vi "输入数据解析.vi"(0 "单个参数补充":dbl, 1 "从板号":dbl=1.0, 2 "主板二维码":string="BNET01", 3 "从板二维码":string="BNET01", 5 "主板引用":refnum<vi>, 7 "从板引用":refnum<vi>, 9 "主板选项":string="三级故障阀值", 11 "枚举":enum16{"主板", "从板"}(ring), 12 "快换":bool caption="快换写入") -> (4 "输出数组":dbl[][](array[numeric]), 6 "数组长度":dbl[](array[numeric]), 8 "循环次数":i32, 10 "命令":u32, 14 "名称":string[](array[string]), 15 "命令序号":u32[](array[numeric]))   [LabVIEW 2013] (continued)
                    n6602 = call "输入分辨率计算-EV05.vi"("1字节?"=FALSE, "数值"=w16869, "分辨率"=0.001) -> ("低字节"=w16871:dbl, "高字节1"=w16872:dbl)  [unwired: 2 in, 5 out]
                  }
                  frame Disabled {
                    w16875 = 255 ("高字节1")
                  }
                }
                n6603 = Build Array(w16868, w16867) -> (w16866:dbl[])
              }
              frame 1 {
                # "电压过低"
                n6604 = disable-structure shown="启用" {
                  disable-tunnel: [w16883 w16886] -> w16879
                  disable-tunnel: [w16882 w16886] -> w16878
                  disable-tunnel: w16876 -> [w16881 _]
                  frame Disabled {
                    n6605 = Unbundle By Name(w16881) -> ("电压过低"=w16880:dbl)
                    n6606 = call "输入分辨率计算-EV05.vi"("1字节?"=FALSE, "数值"=w16880, "分辨率"=0.1) -> ("低字节"=w16882:dbl, "高字节1"=w16883:dbl)  [unwired: 2 in, 5 out]
                  }
                  frame Enabled {
                    w16886 = 255 ("高字节1")
                  }
                }
                n6607 = Build Array(w16879, w16878) -> (w16877:i32[])
              }
              frame 2 {
                # "电压不均衡"
                n6608 = disable-structure shown="启用" {
                  disable-tunnel: [w16894 w16897] -> w16890
                  disable-tunnel: [w16893 w16897] -> w16889
                  disable-tunnel: w16887 -> [w16892 _]
                  frame Disabled {
                    n6609 = Unbundle By Name(w16892) -> ("电压不均衡(V)"=w16891:dbl)
                    n6610 = call "输入分辨率计算-EV05.vi"("1字节?"=FALSE, "数值"=w16891, "分辨率"=0.1) -> ("低字节"=w16893:dbl, "高字节1"=w16894:dbl)  [unwired: 2 in, 5 out]
                  }
                  frame Enabled {
                    w16897 = 255 ("高字节1")
                  }
                }
                n6611 = Build Array(w16890, w16889) -> (w16888:i32[])
              }
              frame 3 {
                # "温度过高"
                n6612 = disable-structure shown="启用" {
                  disable-tunnel: [w16904 255 ("高字节1")] -> w16900
                  disable-tunnel: w16898 -> [w16902 _]
                  frame Disabled {
                    n6613 = Unbundle By Name(w16902) -> ("温度过高"=w16901:dbl)
                    n6614 = call "输入分辨率计算-EV05.vi"("1字节?"=TRUE, "数值"=w16901, "偏移量"=-40.0, "分辨率"=1.0) -> ("高字节1"=w16904:dbl)  [unwired: 1 in, 6 out]
                  }
                  frame Enabled {
                  }
                }
                n6615 = Build Array(w16900) -> (w16899:i32[])
              }
              frame 4 {
                # "温度过低"
                n6616 = disable-structure shown="启用" {
                  disable-tunnel: [w16914 255 ("高字节1")] -> w16910
                  disable-tunnel: w16908 -> [w16912 _]
                  frame Disabled {
                    n6617 = Unbundle By Name(w16912) -> ("温度过低"=w16911:dbl)
                    n6618 = call "输入分辨率计算-EV05.vi"("1字节?"=TRUE, "数值"=w16911, "偏移量"=-40.0, "分辨率"=1.0) -> ("高字节1"=w16914:dbl)  [unwired: 1 in, 6 out]
                  }
                  frame Enabled {
                  }
                }
                n6619 = Build Array(w16910) -> (w16909:i32[])
              }
              frame 5 {
                # "温度不均衡"
                n6620 = disable-structure shown="启用" {
                  disable-tunnel: [w16923 255 ("高字节1")] -> w16920
                  disable-tunnel: w16918 -> [w16922 _]
                  frame Disabled {
                    n6621 = Unbundle By Name(w16922) -> ("温度不均衡"=w16921:dbl)
                    n6622 = call "输入分辨率计算-EV05.vi"("1字节?"=TRUE, "数值"=w16921, "分辨率"=1.0) -> ("高字节1"=w16923:dbl)  [unwired: 2 in, 6 out]
                  }
                  frame Enabled {
                  }
                }
                n6623 = Build Array(w16920) -> (w16919:i32[])
              }
              frame 6 {
                # "SOC过低"
                n6624 = disable-structure shown="启用" {
                  disable-tunnel: w16929 -> [w16946 _]
                  disable-tunnel: [w16932 w16949] -> w16928
                  disable-tunnel: [w16931 w16949] -> w16927
                  frame Disabled {
                    n6625 = Unbundle By Name(w16946) -> ("SOC过低"=w16945:dbl)
                    n6626 = call "输入分辨率计算-EV05.vi"("1字节?"=FALSE, "数值"=w16945, "分辨率"=0.1) -> ("低字节"=w16934:dbl, "高字节1"=w16935:dbl)  [unwired: 2 in, 5 out]
                    n6627 = call "二进制解析-8.6.vi"("索引"=4, "数值"=0) -> ("低位子数组"=w16938:i32[])  [unwired: 3 out]
                    n6628 = call "二进制解析-8.6.vi"("索引"=4, "数值"=w16935) -> ("低位子数组"=w16941:i32[])  [unwired: 3 out]
                    n6629 = call "二进制解析-8.6.vi"("索引"=4, "数值"=w16934) -> ("低位子数组"=w16939:i32[], "高位子数组"=w16940:i32[])  [unwired: 2 out]
                    n6630 = Insert Into Array(array=w16941, new element=w16940) -> (w16943:i32[])  [unwired: 1 in]
                    n6631 = Insert Into Array(array=w16939, new element=w16938) -> (w16937:i32[])  [unwired: 1 in]
                    n6632 = call "数值二进制转十进制-8.6.vi"("子数组"=w16937) -> ("十进制数值"=w16932:i32)  [unwired: 4 out]
                    n6633 = call "数值二进制转十进制-8.6.vi"("子数组"=w16943) -> ("十进制数值"=w16931:i32)  [unwired: 4 out]
                  }
                  frame Enabled {
                    w16949 = 255 ("高字节1")
                  }
                }
                n6634 = Build Array(w16927, w16928) -> (w16930:i32[])
              }
            }
            n6635 = Insert Into Array(array=w16861, new element=w16860) -> (w16862:dbl[])  [unwired: 1 in]
          }
          n6636 = Build Array(w16855) -> (w16854:dbl[][])
        }
        frame "电压过低" {
          n6637 = Unbundle By Name(w16954) -> ("一级故障(从板)"=w16955:refnum<vi>)
          n6638 = property class="Clust (严格)"(reference=w16955) -> ("Value"=w16953:T8)  [unwired: 1 in, 2 out]
          n6639 = for {
            N: 7 -> [_]
            tunnel: w16953 -> [w16965]
            shift-right: [w16964] -> w16957
            shift-left: dbl[] [] -> [w16963]
            i -> [w16966]
            n6640 = case shown="1" w16966 {
              tunnel: w16965 -> [w16967 w16978 w16989 w17000 w17010 w17020 w17031]
              tunnel: [w16968 w16979 w16990 w17001 w17011 w17021 w17032] -> w16962
              frame 0, Default {
                # "电压过高"
                n6641 = disable-structure shown="启用" {
                  disable-tunnel: [w16974 w16977] -> w16970
                  disable-tunnel: [w16973 w16977] -> w16969
                  disable-tunnel: w16967 -> [w16972 _]
                  frame Disabled {
                    n6642 = Unbundle By Name(w16972) -> ("电压过高"=w16971:dbl)
                    n6643 = call "输入分辨率计算-EV05.vi"("1字节?"=FALSE, "数值"=w16971, "分辨率"=0.1) -> ("低字节"=w16973:dbl, "高字节1"=w16974:dbl)  [unwired: 2 in, 5 out]
                  }
                  frame Enabled {
                    w16977 = 255 ("高字节1")
                  }
                }
                n6644 = Build Array(w16970, w16969) -> (w16968:i32[])
              }
              frame 1 {
                # "电压过低"
                n6645 = disable-structure shown="启用" {
                  disable-tunnel: [w16985 w16988] -> w16981
                  disable-tunnel: [w16984 w16988] -> w16980
                  disable-tunnel: w16978 -> [w16983 _]
                  frame Enabled {
                    n6646 = Unbundle By Name(w16983) -> ("电压过低"=w16982:dbl)
                    n6647 = call "输入分辨率计算-EV05.vi"("1字节?"=FALSE, "数值"=w16982, "分辨率"=0.001) -> ("低字节"=w16984:dbl, "高字节1"=w16985:dbl)  [unwired: 2 in, 5 out]
                  }
                  frame Disabled {
                    w16988 = 255 ("高字节1")
                  }
                }
                n6648 = Build Array(w16981, w16980) -> (w16979:dbl[])
              }
              frame 2 {
                # "电压不均衡"
                n6649 = disable-structure shown="启用" {
                  disable-tunnel: [w16996 w16999] -> w16992
                  disable-tunnel: [w16995 w16999] -> w16991
                  disable-tunnel: w16989 -> [w16994 _]
                  frame Disabled {
                    n6650 = Unbundle By Name(w16994) -> ("电压不均衡(V)"=w16993:dbl)
                    n6651 = call "输入分辨率计算-EV05.vi"("1字节?"=FALSE, "数值"=w16993, "分辨率"=0.1) -> ("低字节"=w16995:dbl, "高字节1"=w16996:dbl)  [unwired: 2 in, 5 out]
                  }
                  frame Enabled {
                    w16999 = 255 ("高字节1")
                  }
                }
                n6652 = Build Array(w16992, w16991) -> (w16990:i32[])
              }
              frame 3 {
                # "温度过高"
                n6653 = disable-structure shown="启用" {
                  disable-tunnel: [w17006 255 ("高字节1")] -> w17002
                  disable-tunnel: w17000 -> [w17004 _]
                  frame Disabled {
                    n6654 = Unbundle By Name(w17004) -> ("温度过高"=w17003:dbl)
                    n6655 = call "输入分辨率计算-EV05.vi"("1字节?"=TRUE, "数值"=w17003, "偏移量"=-40.0, "分辨率"=1.0) -> ("高字节1"=w17006:dbl)  [unwired: 1 in, 6 out]
                  }
                  frame Enabled {
                  }
                }
                n6656 = Build Array(w17002) -> (w17001:i32[])
              }
              frame 4 {
                # "温度过低"
                n6657 = disable-structure shown="启用" {
                  disable-tunnel: [w17016 255 ("高字节1")] -> w17012
                  disable-tunnel: w17010 -> [w17014 _]
                  frame Disabled {
                    n6658 = Unbundle By Name(w17014) -> ("温度过低"=w17013:dbl)
                    n6659 = call "输入分辨率计算-EV05.vi"("1字节?"=TRUE, "数值"=w17013, "偏移量"=-40.0, "分辨率"=1.0) -> ("高字节1"=w17016:dbl)  [unwired: 1 in, 6 out]
                  }
                  frame Enabled {
                  }
                }
                n6660 = Build Array(w17012) -> (w17011:i32[])
              }
              frame 5 {
                # "温度不均衡"
                n6661 = disable-structure shown="启用" {
                  disable-tunnel: [w17025 255 ("高字节1")] -> w17022
                  disable-tunnel: w17020 -> [w17024 _]
                  frame Disabled {
                    n6662 = Unbundle By Name(w17024) -> ("温度不均衡"=w17023:dbl)
                    n6663 = call "输入分辨率计算-EV05.vi"("1字节?"=TRUE, "数值"=w17023, "分辨率"=1.0) -> ("高字节1"=w17025:dbl)  [unwired: 2 in, 6 out]
                  }
                  frame Enabled {
                  }
                }
                n6664 = Build Array(w17022) -> (w17021:i32[])
              }
              frame 6 {
                # "SOC过低"
                n6665 = disable-structure shown="启用" {
                  disable-tunnel: w17031 -> [w17048 _]
                  disable-tunnel: [w17034 w17051] -> w17030
                  disable-tunnel: [w17033 w17051] -> w17029
                  frame Disabled {
                    n6666 = Unbundle By Name(w17048) -> ("SOC过低"=w17047:dbl)
                    n6667 = call "输入分辨率计算-EV05.vi"("1字节?"=FALSE, "数值"=w17047, "分辨率"=0.1) -> ("低字节"=w17036:dbl, "高字节1"=w17037:dbl)  [unwired: 2 in, 5 out]
                    n6668 = call "二进制解析-8.6.vi"("索引"=4, "数值"=0) -> ("低位子数组"=w17040:i32[])  [unwired: 3 out]
                    n6669 = call "二进制解析-8.6.vi"("索引"=4, "数值"=w17037) -> ("低位子数组"=w17043:i32[])  [unwired: 3 out]
                    n6670 = call "二进制解析-8.6.vi"("索引"=4, "数值"=w17036) -> ("低位子数组"=w17041:i32[], "高位子数组"=w17042:i32[])  [unwired: 2 out]
                    n6671 = Insert Into Array(array=w17043, new element=w17042) -> (w17045:i32[])  [unwired: 1 in]
                    n6672 = Insert Into Array(array=w17041, new element=w17040) -> (w17039:i32[])  [unwired: 1 in]
                    n6673 = call "数值二进制转十进制-8.6.vi"("子数组"=w17039) -> ("十进制数值"=w17034:i32)  [unwired: 4 out]
                    n6674 = call "数值二进制转十进制-8.6.vi"("子数组"=w17045) -> ("十进制数值"=w17033:i32)  [unwired: 4 out]
                  }
                  frame Enabled {
                    w17051 = 255 ("高字节1")
                  }
                }
                n6675 = Build Array(w17029, w17030) -> (w17032:i32[])
              }
            }
            n6676 = Insert Into Array(array=w16963, new element=w16962) -> (w16964:dbl[])  [unwired: 1 in]
          }
          n6677 = Build Array(w16957) -> (w16956:dbl[][])
        }
        frame "电压过低(2)" {
          n6678 = Unbundle By Name(w17056) -> ("二级故障(从板)"=w17057:refnum<vi>)
          n6679 = property class="Clust (严格)"(reference=w17057) -> ("Value"=w17055:T8)  [unwired: 1 in, 2 out]
          n6680 = for {
            N: 7 -> [_]
            tunnel: w17055 -> [w17067]
            shift-right: [w17066] -> w17059
            shift-left: dbl[] [] -> [w17065]
            i -> [w17068]
            n6681 = case shown="1" w17068 {
              tunnel: w17067 -> [w17069 w17080 w17091 w17102 w17112 w17122 w17133]
              tunnel: [w17070 w17081 w17092 w17103 w17113 w17123 w17134] -> w17064
              frame 0, Default {
                # "电压过高"
                n6682 = disable-structure shown="启用" {
                  disable-tunnel: [w17076 w17079] -> w17072
                  disable-tunnel: [w17075 w17079] -> w17071
                  disable-tunnel: w17069 -> [w17074 _]
                  frame Disabled {
                    n6683 = Unbundle By Name(w17074) -> ("电压过高"=w17073:dbl)
                    n6684 = call "输入分辨率计算-EV05.vi"("1字节?"=FALSE, "数值"=w17073, "分辨率"=0.1) -> ("低字节"=w17075:dbl, "高字节1"=w17076:dbl)  [unwired: 2 in, 5 out]
                  }
                  frame Enabled {
                    w17079 = 255 ("高字节1")
                  }
                }
                n6685 = Build Array(w17072, w17071) -> (w17070:i32[])
              }
              frame 1 {
                # "电压过低"
                n6686 = disable-structure shown="启用" {
                  disable-tunnel: [w17087 w17090] -> w17083
                  disable-tunnel: [w17086 w17090] -> w17082
                  disable-tunnel: w17080 -> [w17085 _]
                  frame Enabled {
                    n6687 = Unbundle By Name(w17085) -> ("电压过低"=w17084:dbl)
                    n6688 = call "输入分辨率计算-EV05.vi"("1字节?"=FALSE, "数值"=w17084, "分辨率"=0.001) -> ("低字节"=w17086:dbl, "高字节1"=w17087:dbl)  [unwired: 2 in, 5 out]
                  }
                  frame Disabled {
                    w17090 = 255 ("高字节1")
                  }
                }
                n6689 = Build Array(w17083, w17082) -> (w17081:dbl[])
              }
              frame 2 {
                # "电压不均衡"
                n6690 = disable-structure shown="启用" {
                  disable-tunnel: [w17098 w17101] -> w17094
                  disable-tunnel: [w17097 w17101] -> w17093
                  disable-tunnel: w17091 -> [w17096 _]
                  frame Disabled {
                    n6691 = Unbundle By Name(w17096) -> ("电压不均衡(V)"=w17095:dbl)
                    n6692 = call "输入分辨率计算-EV05.vi"("1字节?"=FALSE, "数值"=w17095, "分辨率"=0.1) -> ("低字节"=w17097:dbl, "高字节1"=w17098:dbl)  [unwired: 2 in, 5 out]
                  }
                  frame Enabled {
                    w17101 = 255 ("高字节1")
                  }
                }
                n6693 = Build Array(w17094, w17093) -> (w17092:i32[])
              }
              frame 3 {
                # "温度过高"
                n6694 = disable-structure shown="启用" {
                  disable-tunnel: [w17108 255 ("高字节1")] -> w17104
                  disable-tunnel: w17102 -> [w17106 _]
                  frame Disabled {
                    n6695 = Unbundle By Name(w17106) -> ("温度过高"=w17105:dbl)
                    n6696 = call "输入分辨率计算-EV05.vi"("1字节?"=TRUE, "数值"=w17105, "偏移量"=-40.0, "分辨率"=1.0) -> ("高字节1"=w17108:dbl)  [unwired: 1 in, 6 out]
                  }
                  frame Enabled {
                  }
                }
                n6697 = Build Array(w17104) -> (w17103:i32[])
              }
              frame 4 {
                # "温度过低"
                n6698 = disable-structure shown="启用" {
                  disable-tunnel: [w17118 255 ("高字节1")] -> w17114
                  disable-tunnel: w17112 -> [w17116 _]
                  frame Disabled {
                    n6699 = Unbundle By Name(w17116) -> ("温度过低"=w17115:dbl)
                    n6700 = call "输入分辨率计算-EV05.vi"("1字节?"=TRUE, "数值"=w17115, "偏移量"=-40.0, "分辨率"=1.0) -> ("高字节1"=w17118:dbl)  [unwired: 1 in, 6 out]
                  }
                  frame Enabled {
                  }
                }
                n6701 = Build Array(w17114) -> (w17113:i32[])
              }
              frame 5 {
                # "温度不均衡"
                n6702 = disable-structure shown="启用" {
                  disable-tunnel: [w17127 255 ("高字节1")] -> w17124
                  disable-tunnel: w17122 -> [w17126 _]
                  frame Disabled {
                    n6703 = Unbundle By Name(w17126) -> ("温度不均衡"=w17125:dbl)
                    n6704 = call "输入分辨率计算-EV05.vi"("1字节?"=TRUE, "数值"=w17125, "分辨率"=1.0) -> ("高字节1"=w17127:dbl)  [unwired: 2 in, 6 out]
                  }
                  frame Enabled {
                  }
                }
                n6705 = Build Array(w17124) -> (w17123:i32[])
              }
              frame 6 {
                # "SOC过低"
                n6706 = disable-structure shown="启用" {
                  disable-tunnel: w17133 -> [w17150 _]
                  disable-tunnel: [w17136 w17153] -> w17132
                  disable-tunnel: [w17135 w17153] -> w17131
                  frame Disabled {
                    n6707 = Unbundle By Name(w17150) -> ("SOC过低"=w17149:dbl)
                    n6708 = call "输入分辨率计算-EV05.vi"("1字节?"=FALSE, "数值"=w17149, "分辨率"=0.1) -> ("低字节"=w17138:dbl, "高字节1"=w17139:dbl)  [unwired: 2 in, 5 out]
                    n6709 = call "二进制解析-8.6.vi"("索引"=4, "数值"=0) -> ("低位子数组"=w17142:i32[])  [unwired: 3 out]
                    n6710 = call "二进制解析-8.6.vi"("索引"=4, "数值"=w17139) -> ("低位子数组"=w17145:i32[])  [unwired: 3 out]
                    n6711 = call "二进制解析-8.6.vi"("索引"=4, "数值"=w17138) -> ("低位子数组"=w17143:i32[], "高位子数组"=w17144:i32[])  [unwired: 2 out]
                    n6712 = Insert Into Array(array=w17145, new element=w17144) -> (w17147:i32[])  [unwired: 1 in]
                    n6713 = Insert Into Array(array=w17143, new element=w17142) -> (w17141:i32[])  [unwired: 1 in]
                    n6714 = call "数值二进制转十进制-8.6.vi"("子数组"=w17141) -> ("十进制数值"=w17136:i32)  [unwired: 4 out]
                    n6715 = call "数值二进制转十进制-8.6.vi"("子数组"=w17147) -> ("十进制数值"=w17135:i32)  [unwired: 4 out]
                  }
                  frame Enabled {
                    w17153 = 255 ("高字节1")
                  }
                }
                n6716 = Build Array(w17131, w17132) -> (w17134:i32[])
              }
            }
            n6717 = Insert Into Array(array=w17065, new element=w17064) -> (w17066:dbl[])  [unwired: 1 in]
          }
          n6718 = Build Array(w17059) -> (w17058:dbl[][])
        }
        frame "电压过低(3)" {
          n6719 = Unbundle By Name(w17158) -> ("三级故障(从板)"=w17159:refnum<vi>)
          n6720 = property class="Clust (严格)"(reference=w17159) -> ("Value"=w17157:T8)  [unwired: 1 in, 2 out]
          n6721 = for {
            N: 7 -> [_]
            tunnel: w17157 -> [w17169]
            shift-right: [w17168] -> w17161
            shift-left: dbl[] [] -> [w17167]
            i -> [w17170]
            n6722 = case shown="1" w17170 {
              tunnel: w17169 -> [w17171 w17182 w17193 w17204 w17214 w17224 w17235]
              tunnel: [w17172 w17183 w17194 w17205 w17215 w17225 w17236] -> w17166
              frame 0, Default {
                # "电压过高"
                n6723 = disable-structure shown="启用" {
                  disable-tunnel: [w17178 w17181] -> w17174
                  disable-tunnel: [w17177 w17181] -> w17173
                  disable-tunnel: w17171 -> [w17176 _]
                  frame Disabled {
                    n6724 = Unbundle By Name(w17176) -> ("电压过高"=w17175:dbl)
                    n6725 = call "输入分辨率计算-EV05.vi"("1字节?"=FALSE, "数值"=w17175, "分辨率"=0.1) -> ("低字节"=w17177:dbl, "高字节1"=w17178:dbl)  [unwired: 2 in, 5 out]
                  }
                  frame Enabled {
                    w17181 = 255 ("高字节1")
                  }
                }
                n6726 = Build Array(w17174, w17173) -> (w17172:i32[])
              }
              frame 1 {
                # "电压过低"
                n6727 = disable-structure shown="启用" {
                  disable-tunnel: [w17189 w17192] -> w17185
                  disable-tunnel: [w17188 w17192] -> w17184
                  disable-tunnel: w17182 -> [w17187 _]
                  frame Enabled {
                    n6728 = Unbundle By Name(w17187) -> ("电压过低"=w17186:dbl)
                    n6729 = call "输入分辨率计算-EV05.vi"("1字节?"=FALSE, "数值"=w17186, "分辨率"=0.001) -> ("低字节"=w17188:dbl, "高字节1"=w17189:dbl)  [unwired: 2 in, 5 out]
                  }
                  frame Disabled {
                    w17192 = 255 ("高字节1")
                  }
                }
                n6730 = Build Array(w17185, w17184) -> (w17183:dbl[])
              }
              frame 2 {
                # "电压不均衡"
                n6731 = disable-structure shown="启用" {
                  disable-tunnel: [w17200 w17203] -> w17196
                  disable-tunnel: [w17199 w17203] -> w17195
                  disable-tunnel: w17193 -> [w17198 _]
                  frame Disabled {
                    n6732 = Unbundle By Name(w17198) -> ("电压不均衡(V)"=w17197:dbl)
                    n6733 = call "输入分辨率计算-EV05.vi"("1字节?"=FALSE, "数值"=w17197, "分辨率"=0.1) -> ("低字节"=w17199:dbl, "高字节1"=w17200:dbl)  [unwired: 2 in, 5 out]
                  }
                  frame Enabled {
                    w17203 = 255 ("高字节1")
                  }
                }
                n6734 = Build Array(w17196, w17195) -> (w17194:i32[])
              }
              frame 3 {
                # "温度过高"
                n6735 = disable-structure shown="启用" {
                  disable-tunnel: [w17210 255 ("高字节1")] -> w17206
                  disable-tunnel: w17204 -> [w17208 _]
                  frame Disabled {
                    n6736 = Unbundle By Name(w17208) -> ("温度过高"=w17207:dbl)
                    n6737 = call "输入分辨率计算-EV05.vi"("1字节?"=TRUE, "数值"=w17207, "偏移量"=-40.0, "分辨率"=1.0) -> ("高字节1"=w17210:dbl)  [unwired: 1 in, 6 out]
                  }
                  frame Enabled {
                  }
                }
                n6738 = Build Array(w17206) -> (w17205:i32[])
              }
              frame 4 {
                # "温度过低"
                n6739 = disable-structure shown="启用" {
                  disable-tunnel: [w17220 255 ("高字节1")] -> w17216
                  disable-tunnel: w17214 -> [w17218 _]
                  frame Disabled {
                    n6740 = Unbundle By Name(w17218) -> ("温度过低"=w17217:dbl)
                    n6741 = call "输入分辨率计算-EV05.vi"("1字节?"=TRUE, "数值"=w17217, "偏移量"=-40.0, "分辨率"=1.0) -> ("高字节1"=w17220:dbl)  [unwired: 1 in, 6 out]
                  }
                  frame Enabled {
                  }
                }
                n6742 = Build Array(w17216) -> (w17215:i32[])
              }
              frame 5 {
                # "温度不均衡"
                n6743 = disable-structure shown="启用" {
                  disable-tunnel: [w17229 255 ("高字节1")] -> w17226
                  disable-tunnel: w17224 -> [w17228 _]
                  frame Disabled {
                    n6744 = Unbundle By Name(w17228) -> ("温度不均衡"=w17227:dbl)
                    n6745 = call "输入分辨率计算-EV05.vi"("1字节?"=TRUE, "数值"=w17227, "分辨率"=1.0) -> ("高字节1"=w17229:dbl)  [unwired: 2 in, 6 out]
                  }
                  frame Enabled {
                  }
                }
                n6746 = Build Array(w17226) -> (w17225:i32[])
              }
              frame 6 {
                # "SOC过低"
                n6747 = disable-structure shown="启用" {
                  disable-tunnel: w17235 -> [w17252 _]
                  disable-tunnel: [w17238 w17255] -> w17234
                  disable-tunnel: [w17237 w17255] -> w17233
                  frame Disabled {
                    n6748 = Unbundle By Name(w17252) -> ("SOC过低"=w17251:dbl)
                    n6749 = call "输入分辨率计算-EV05.vi"("1字节?"=FALSE, "数值"=w17251, "分辨率"=0.1) -> ("低字节"=w17240:dbl, "高字节1"=w17241:dbl)  [unwired: 2 in, 5 out]
                    n6750 = call "二进制解析-8.6.vi"("索引"=4, "数值"=0) -> ("低位子数组"=w17244:i32[])  [unwired: 3 out]
                    n6751 = call "二进制解析-8.6.vi"("索引"=4, "数值"=w17241) -> ("低位子数组"=w17247:i32[])  [unwired: 3 out]
                    n6752 = call "二进制解析-8.6.vi"("索引"=4, "数值"=w17240) -> ("低位子数组"=w17245:i32[], "高位子数组"=w17246:i32[])  [unwired: 2 out]
                    n6753 = Insert Into Array(array=w17247, new element=w17246) -> (w17249:i32[])  [unwired: 1 in]
                    n6754 = Insert Into Array(array=w17245, new element=w17244) -> (w17243:i32[])  [unwired: 1 in]
                    n6755 = call "数值二进制转十进制-8.6.vi"("子数组"=w17243) -> ("十进制数值"=w17238:i32)  [unwired: 4 out]
                    n6756 = call "数值二进制转十进制-8.6.vi"("子数组"=w17249) -> ("十进制数值"=w17237:i32)  [unwired: 4 out]
                  }
                  frame Enabled {
                    w17255 = 255 ("高字节1")
                  }
                }
                n6757 = Build Array(w17233, w17234) -> (w17236:i32[])
              }
            }
            n6758 = Insert Into Array(array=w17167, new element=w17166) -> (w17168:dbl[])  [unwired: 1 in]
          }
          n6759 = Build Array(w17161) -> (w17160:dbl[][])
        }
        frame "电压不均衡" {
          n6760 = Unbundle By Name(w17260) -> ("一级故障(从板)"=w17261:refnum<vi>)
          n6761 = property class="Clust (严格)"(reference=w17261) -> ("Value"=w17259:T8)  [unwired: 1 in, 2 out]
          n6762 = for {
            N: 7 -> [_]
            tunnel: w17259 -> [w17271]
            shift-right: [w17270] -> w17263
            shift-left: dbl[] [] -> [w17269]
            i -> [w17272]
            n6763 = case shown="3" w17272 {
              tunnel: w17271 -> [w17273 w17284 w17295 w17306 w17316 w17326 w17337]
              tunnel: [w17274 w17285 w17296 w17307 w17317 w17327 w17338] -> w17268
              frame 0, Default {
                # "电压过高"
                n6764 = disable-structure shown="启用" {
                  disable-tunnel: [w17280 w17283] -> w17276
                  disable-tunnel: [w17279 w17283] -> w17275
                  disable-tunnel: w17273 -> [w17278 _]
                  frame Disabled {
                    n6765 = Unbundle By Name(w17278) -> ("电压过高"=w17277:dbl)
                    n6766 = call "输入分辨率计算-EV05.vi"("1字节?"=FALSE, "数值"=w17277, "分辨率"=0.1) -> ("低字节"=w17279:dbl, "高字节1"=w17280:dbl)  [unwired: 2 in, 5 out]
                  }
                  frame Enabled {
                    w17283 = 255 ("高字节1")
                  }
                }
                n6767 = Build Array(w17276, w17275) -> (w17274:i32[])
              }
              frame 1 {
                # "电压过低"
                n6768 = disable-structure shown="启用" {
                  disable-tunnel: [w17291 w17294] -> w17287
                  disable-tunnel: [w17290 w17294] -> w17286
                  disable-tunnel: w17284 -> [w17289 _]
                  frame Disabled {
                    n6769 = Unbundle By Name(w17289) -> ("电压过低"=w17288:dbl)
                    n6770 = call "输入分辨率计算-EV05.vi"("1字节?"=FALSE, "数值"=w17288, "分辨率"=0.1) -> ("低字节"=w17290:dbl, "高字节1"=w17291:dbl)  [unwired: 2 in, 5 out]
                  }
                  frame Enabled {
                    w17294 = 255 ("高字节1")
                  }
                }
                n6771 = Build Array(w17287, w17286) -> (w17285:i32[])
              }
              frame 2 {
                # "电压不均衡"
                n6772 = disable-structure shown="启用" {
                  disable-tunnel: [w17302 w17305] -> w17298
                  disable-tunnel: [w17301 w17305] -> w17297
                  disable-tunnel: w17295 -> [w17300 _]
                  frame Enabled {
                    n6773 = Unbundle By Name(w17300) -> ("电压不均衡(V)"=w17299:dbl)
                    n6774 = call "输入分辨率计算-EV05.vi"("1字节?"=FALSE, "数值"=w17299, "分辨率"=0.001) -> ("低字节"=w17301:dbl, "高字节1"=w17302:dbl)  [unwired: 2 in, 5 out]
                  }
                  frame Disabled {
                    w17305 = 255 ("高字节1")
                  }
                }
                n6775 = Build Array(w17298, w17297) -> (w17296:dbl[])
              }
              frame 3 {
                # "温度过高"
                n6776 = disable-structure shown="启用" {
                  disable-tunnel: [w17312 255 ("高字节1")] -> w17308
                  disable-tunnel: w17306 -> [w17310 _]
                  frame Disabled {
                    n6777 = Unbundle By Name(w17310) -> ("温度过高"=w17309:dbl)
                    n6778 = call "输入分辨率计算-EV05.vi"("1字节?"=TRUE, "数值"=w17309, "偏移量"=-40.0, "分辨率"=1.0) -> ("高字节1"=w17312:dbl)  [unwired: 1 in, 6 out]
                  }
                  frame Enabled {
                  }
                }
                n6779 = Build Array(w17308) -> (w17307:i32[])
              }
              frame 4 {
                # "温度过低"
                n6780 = disable-structure shown="启用" {
                  disable-tunnel: [w17322 255 ("高字节1")] -> w17318
                  disable-tunnel: w17316 -> [w17320 _]
                  frame Disabled {
                    n6781 = Unbundle By Name(w17320) -> ("温度过低"=w17319:dbl)
                    n6782 = call "输入分辨率计算-EV05.vi"("1字节?"=TRUE, "数值"=w17319, "偏移量"=-40.0, "分辨率"=1.0) -> ("高字节1"=w17322:dbl)  [unwired: 1 in, 6 out]
                  }
                  frame Enabled {
                  }
                }
                n6783 = Build Array(w17318) -> (w17317:i32[])
              }
              frame 5 {
                # "温度不均衡"
                n6784 = disable-structure shown="启用" {
                  disable-tunnel: [w17331 255 ("高字节1")] -> w17328
                  disable-tunnel: w17326 -> [w17330 _]
                  frame Disabled {
                    n6785 = Unbundle By Name(w17330) -> ("温度不均衡"=w17329:dbl)
                    n6786 = call "输入分辨率计算-EV05.vi"("1字节?"=TRUE, "数值"=w17329, "分辨率"=1.0) -> ("高字节1"=w17331:dbl)  [unwired: 2 in, 6 out]
                  }
                  frame Enabled {
                  }
                }
                n6787 = Build Array(w17328) -> (w17327:i32[])
              }
              frame 6 {
                # "SOC过低"
                n6788 = disable-structure shown="启用" {
                  disable-tunnel: w17337 -> [w17354 _]
                  disable-tunnel: [w17340 w17357] -> w17336
                  disable-tunnel: [w17339 w17357] -> w17335
                  frame Disabled {
                    n6789 = Unbundle By Name(w17354) -> ("SOC过低"=w17353:dbl)
                    n6790 = call "输入分辨率计算-EV05.vi"("1字节?"=FALSE, "数值"=w17353, "分辨率"=0.1) -> ("低字节"=w17342:dbl, "高字节1"=w17343:dbl)  [unwired: 2 in, 5 out]
                    n6791 = call "二进制解析-8.6.vi"("索引"=4, "数值"=0) -> ("低位子数组"=w17346:i32[])  [unwired: 3 out]
                    n6792 = call "二进制解析-8.6.vi"("索引"=4, "数值"=w17343) -> ("低位子数组"=w17349:i32[])  [unwired: 3 out]
                    n6793 = call "二进制解析-8.6.vi"("索引"=4, "数值"=w17342) -> ("低位子数组"=w17347:i32[], "高位子数组"=w17348:i32[])  [unwired: 2 out]
                    n6794 = Insert Into Array(array=w17349, new element=w17348) -> (w17351:i32[])  [unwired: 1 in]
                    n6795 = Insert Into Array(array=w17347, new element=w17346) -> (w17345:i32[])  [unwired: 1 in]
                    n6796 = call "数值二进制转十进制-8.6.vi"("子数组"=w17345) -> ("十进制数值"=w17340:i32)  [unwired: 4 out]
                    n6797 = call "数值二进制转十进制-8.6.vi"("子数组"=w17351) -> ("十进制数值"=w17339:i32)  [unwired: 4 out]
                  }
                  frame Enabled {
                    w17357 = 255 ("高字节1")
                  }
                }
                n6798 = Build Array(w17335, w17336) -> (w17338:i32[])
              }
            }
            n6799 = Insert Into Array(array=w17269, new element=w17268) -> (w17270:dbl[])  [unwired: 1 in]
          }
          n6800 = Build Array(w17263) -> (w17262:dbl[][])
        }
        frame "电压不均衡(2)" {
          n6801 = Unbundle By Name(w17362) -> ("二级故障(从板)"=w17363:refnum<vi>)
          n6802 = property class="Clust (严格)"(reference=w17363) -> ("Value"=w17361:T8)  [unwired: 1 in, 2 out]
          n6803 = for {
            N: 7 -> [_]
            tunnel: w17361 -> [w17373]
            shift-right: [w17372] -> w17365
            shift-left: dbl[] [] -> [w17371]
            i -> [w17374]
            n6804 = case shown="2" w17374 {
              tunnel: w17373 -> [w17375 w17386 w17397 w17408 w17418 w17428 w17439]
              tunnel: [w17376 w17387 w17398 w17409 w17419 w17429 w17440] -> w17370
              frame 0, Default {
                # "电压过高"
                n6805 = disable-structure shown="启用" {
                  disable-tunnel: [w17382 w17385] -> w17378
                  disable-tunnel: [w17381 w17385] -> w17377
                  disable-tunnel: w17375 -> [w17380 _]
                  frame Disabled {
                    n6806 = Unbundle By Name(w17380) -> ("电压过高"=w17379:dbl)
                    n6807 = call "输入分辨率计算-EV05.vi"("1字节?"=FALSE, "数值"=w17379, "分辨率"=0.1) -> ("低字节"=w17381:dbl, "高字节1"=w17382:dbl)  [unwired: 2 in, 5 out]
                  }
                  frame Enabled {
                    w17385 = 255 ("高字节1")
                  }
                }
                n6808 = Build Array(w17378, w17377) -> (w17376:i32[])
              }
              frame 1 {
                # "电压过低"
                n6809 = disable-structure shown="启用" {
                  disable-tunnel: [w17393 w17396] -> w17389
                  disable-tunnel: [w17392 w17396] -> w17388
                  disable-tunnel: w17386 -> [w17391 _]
                  frame Disabled {
                    n6810 = Unbundle By Name(w17391) -> ("电压过低"=w17390:dbl)
                    n6811 = call "输入分辨率计算-EV05.vi"("1字节?"=FALSE, "数值"=w17390, "分辨率"=0.1) -> ("低字节"=w17392:dbl, "高字节1"=w17393:dbl)  [unwired: 2 in, 5 out]
                  }
                  frame Enabled {
                    w17396 = 255 ("高字节1")
                  }
                }
                n6812 = Build Array(w17389, w17388) -> (w17387:i32[])
              }
              frame 2 {
                # "电压不均衡"
                n6813 = disable-structure shown="启用" {
                  disable-tunnel: [w17404 w17407] -> w17400
                  disable-tunnel: [w17403 w17407] -> w17399
                  disable-tunnel: w17397 -> [w17402 _]
                  frame Enabled {
                    n6814 = Unbundle By Name(w17402) -> ("电压不均衡(V)"=w17401:dbl)
                    n6815 = call "输入分辨率计算-EV05.vi"("1字节?"=FALSE, "数值"=w17401, "分辨率"=0.001) -> ("低字节"=w17403:dbl, "高字节1"=w17404:dbl)  [unwired: 2 in, 5 out]
                  }
                  frame Disabled {
                    w17407 = 255 ("高字节1")
                  }
                }
                n6816 = Build Array(w17400, w17399) -> (w17398:dbl[])
              }
              frame 3 {
                # "温度过高"
                n6817 = disable-structure shown="启用" {
                  disable-tunnel: [w17414 255 ("高字节1")] -> w17410
                  disable-tunnel: w17408 -> [w17412 _]
                  frame Disabled {
                    n6818 = Unbundle By Name(w17412) -> ("温度过高"=w17411:dbl)
                    n6819 = call "输入分辨率计算-EV05.vi"("1字节?"=TRUE, "数值"=w17411, "偏移量"=-40.0, "分辨率"=1.0) -> ("高字节1"=w17414:dbl)  [unwired: 1 in, 6 out]
                  }
                  frame Enabled {
                  }
                }
                n6820 = Build Array(w17410) -> (w17409:i32[])
              }
              frame 4 {
                # "温度过低"
                n6821 = disable-structure shown="启用" {
                  disable-tunnel: [w17424 255 ("高字节1")] -> w17420
                  disable-tunnel: w17418 -> [w17422 _]
                  frame Disabled {
                    n6822 = Unbundle By Name(w17422) -> ("温度过低"=w17421:dbl)
                    n6823 = call "输入分辨率计算-EV05.vi"("1字节?"=TRUE, "数值"=w17421, "偏移量"=-40.0, "分辨率"=1.0) -> ("高字节1"=w17424:dbl)  [unwired: 1 in, 6 out]
                  }
                  frame Enabled {
                  }
                }
                n6824 = Build Array(w17420) -> (w17419:i32[])
              }
              frame 5 {
                # "温度不均衡"
                n6825 = disable-structure shown="启用" {
                  disable-tunnel: [w17433 255 ("高字节1")] -> w17430
                  disable-tunnel: w17428 -> [w17432 _]
                  frame Disabled {
                    n6826 = Unbundle By Name(w17432) -> ("温度不均衡"=w17431:dbl)
                    n6827 = call "输入分辨率计算-EV05.vi"("1字节?"=TRUE, "数值"=w17431, "分辨率"=1.0) -> ("高字节1"=w17433:dbl)  [unwired: 2 in, 6 out]
                  }
                  frame Enabled {
                  }
                }
                n6828 = Build Array(w17430) -> (w17429:i32[])
              }
              frame 6 {
                # "SOC过低"
                n6829 = disable-structure shown="启用" {
                  disable-tunnel: w17439 -> [w17456 _]
                  disable-tunnel: [w17442 w17459] -> w17438
                  disable-tunnel: [w17441 w17459] -> w17437
                  frame Disabled {
                    n6830 = Unbundle By Name(w17456) -> ("SOC过低"=w17455:dbl)
                    n6831 = call "输入分辨率计算-EV05.vi"("1字节?"=FALSE, "数值"=w17455, "分辨率"=0.1) -> ("低字节"=w17444:dbl, "高字节1"=w17445:dbl)  [unwired: 2 in, 5 out]
                    n6832 = call "二进制解析-8.6.vi"("索引"=4, "数值"=0) -> ("低位子数组"=w17448:i32[])  [unwired: 3 out]
                    n6833 = call "二进制解析-8.6.vi"("索引"=4, "数值"=w17445) -> ("低位子数组"=w17451:i32[])  [unwired: 3 out]
                    n6834 = call "二进制解析-8.6.vi"("索引"=4, "数值"=w17444) -> ("低位子数组"=w17449:i32[], "高位子数组"=w17450:i32[])  [unwired: 2 out]
                    n6835 = Insert Into Array(array=w17451, new element=w17450) -> (w17453:i32[])  [unwired: 1 in]
                    n6836 = Insert Into Array(array=w17449, new element=w17448) -> (w17447:i32[])  [unwired: 1 in]
                    n6837 = call "数值二进制转十进制-8.6.vi"("子数组"=w17447) -> ("十进制数值"=w17442:i32)  [unwired: 4 out]
                    n6838 = call "数值二进制转十进制-8.6.vi"("子数组"=w17453) -> ("十进制数值"=w17441:i32)  [unwired: 4 out]
                  }
                  frame Enabled {
                    w17459 = 255 ("高字节1")
                  }
                }
                n6839 = Build Array(w17437, w17438) -> (w17440:i32[])
              }
            }
            n6840 = Insert Into Array(array=w17371, new element=w17370) -> (w17372:dbl[])  [unwired: 1 in]
          }
          n6841 = Build Array(w17365) -> (w17364:dbl[][])
        }
        frame "电压不均衡(3)" {
          n6842 = Unbundle By Name(w17464) -> ("三级故障(从板)"=w17465:refnum<vi>)
          n6843 = property class="Clust (严格)"(reference=w17465) -> ("Value"=w17463:T8)  [unwired: 1 in, 2 out]
          n6844 = for {
            N: 7 -> [_]
            tunnel: w17463 -> [w17475]
            shift-right: [w17474] -> w17467
            shift-left: dbl[] [] -> [w17473]
            i -> [w17476]
            n6845 = case shown="2" w17476 {
              tunnel: w17475 -> [w17477 w17488 w17499 w17510 w17520 w17530 w17541]
              tunnel: [w17478 w17489 w17500 w17511 w17521 w17531 w17542] -> w17472
              frame 0, Default {
                # "电压过高"
                n6846 = disable-structure shown="启用" {
                  disable-tunnel: [w17484 w17487] -> w17480
                  disable-tunnel: [w17483 w17487] -> w17479
                  disable-tunnel: w17477 -> [w17482 _]
                  frame Disabled {
                    n6847 = Unbundle By Name(w17482) -> ("电压过高"=w17481:dbl)
                    n6848 = call "输入分辨率计算-EV05.vi"("1字节?"=FALSE, "数值"=w17481, "分辨率"=0.1) -> ("低字节"=w17483:dbl, "高字节1"=w17484:dbl)  [unwired: 2 in, 5 out]
                  }
                  frame Enabled {
                    w17487 = 255 ("高字节1")
                  }
                }
                n6849 = Build Array(w17480, w17479) -> (w17478:i32[])
              }
              frame 1 {
                # "电压过低"
                n6850 = disable-structure shown="启用" {
                  disable-tunnel: [w17495 w17498] -> w17491
                  disable-tunnel: [w17494 w17498] -> w17490
                  disable-tunnel: w17488 -> [w17493 _]
                  frame Disabled {
                    n6851 = Unbundle By Name(w17493) -> ("电压过低"=w17492:dbl)
                    n6852 = call "输入分辨率计算-EV05.vi"("1字节?"=FALSE, "数值"=w17492, "分辨率"=0.1) -> ("低字节"=w17494:dbl, "高字节1"=w17495:dbl)  [unwired: 2 in, 5 out]
                  }
                  frame Enabled {
                    w17498 = 255 ("高字节1")
                  }
                }
                n6853 = Build Array(w17491, w17490) -> (w17489:i32[])
              }
              frame 2 {
                # "电压不均衡"
                n6854 = disable-structure shown="启用" {
                  disable-tunnel: [w17506 w17509] -> w17502
                  disable-tunnel: [w17505 w17509] -> w17501
                  disable-tunnel: w17499 -> [w17504 _]
                  frame Enabled {
                    n6855 = Unbundle By Name(w17504) -> ("电压不均衡(V)"=w17503:dbl)
                    n6856 = call "输入分辨率计算-EV05.vi"("1字节?"=FALSE, "数值"=w17503, "分辨率"=0.001) -> ("低字节"=w17505:dbl, "高字节1"=w17506:dbl)  [unwired: 2 in, 5 out]
                  }
                  frame Disabled {
                    w17509 = 255 ("高字节1")
                  }
                }
                n6857 = Build Array(w17502, w17501) -> (w17500:dbl[])
              }
              frame 3 {
                # "温度过高"
                n6858 = disable-structure shown="启用" {
                  disable-tunnel: [w17516 255 ("高字节1")] -> w17512
                  disable-tunnel: w17510 -> [w17514 _]
                  frame Disabled {
                    n6859 = Unbundle By Name(w17514) -> ("温度过高"=w17513:dbl)
                    n6860 = call "输入分辨率计算-EV05.vi"("1字节?"=TRUE, "数值"=w17513, "偏移量"=-40.0, "分辨率"=1.0) -> ("高字节1"=w17516:dbl)  [unwired: 1 in, 6 out]
                  }
                  frame Enabled {
                  }
                }
                n6861 = Build Array(w17512) -> (w17511:i32[])
              }
              frame 4 {
                # "温度过低"
                n6862 = disable-structure shown="启用" {
                  disable-tunnel: [w17526 255 ("高字节1")] -> w17522
                  disable-tunnel: w17520 -> [w17524 _]
                  frame Disabled {
                    n6863 = Unbundle By Name(w17524) -> ("温度过低"=w17523:dbl)
                    n6864 = call "输入分辨率计算-EV05.vi"("1字节?"=TRUE, "数值"=w17523, "偏移量"=-40.0, "分辨率"=1.0) -> ("高字节1"=w17526:dbl)  [unwired: 1 in, 6 out]
                  }
                  frame Enabled {
                  }
                }
                n6865 = Build Array(w17522) -> (w17521:i32[])
              }
              frame 5 {
                # "温度不均衡"
                n6866 = disable-structure shown="启用" {
                  disable-tunnel: [w17535 255 ("高字节1")] -> w17532
                  disable-tunnel: w17530 -> [w17534 _]
                  frame Disabled {
                    n6867 = Unbundle By Name(w17534) -> ("温度不均衡"=w17533:dbl)
                    n6868 = call "输入分辨率计算-EV05.vi"("1字节?"=TRUE, "数值"=w17533, "分辨率"=1.0) -> ("高字节1"=w17535:dbl)  [unwired: 2 in, 6 out]
                  }
                  frame Enabled {
                  }
                }
                n6869 = Build Array(w17532) -> (w17531:i32[])
              }
              frame 6 {
                # "SOC过低"
                n6870 = disable-structure shown="启用" {
                  disable-tunnel: w17541 -> [w17558 _]
                  disable-tunnel: [w17544 w17561] -> w17540
                  disable-tunnel: [w17543 w17561] -> w17539
                  frame Disabled {
                    n6871 = Unbundle By Name(w17558) -> ("SOC过低"=w17557:dbl)
                    n6872 = call "输入分辨率计算-EV05.vi"("1字节?"=FALSE, "数值"=w17557, "分辨率"=0.1) -> ("低字节"=w17546:dbl, "高字节1"=w17547:dbl)  [unwired: 2 in, 5 out]
                    n6873 = call "二进制解析-8.6.vi"("索引"=4, "数值"=0) -> ("低位子数组"=w17550:i32[])  [unwired: 3 out]
                    n6874 = call "二进制解析-8.6.vi"("索引"=4, "数值"=w17547) -> ("低位子数组"=w17553:i32[])  [unwired: 3 out]
                    n6875 = call "二进制解析-8.6.vi"("索引"=4, "数值"=w17546) -> ("低位子数组"=w17551:i32[], "高位子数组"=w17552:i32[])  [unwired: 2 out]
                    n6876 = Insert Into Array(array=w17553, new element=w17552) -> (w17555:i32[])  [unwired: 1 in]
                    n6877 = Insert Into Array(array=w17551, new element=w17550) -> (w17549:i32[])  [unwired: 1 in]
                    n6878 = call "数值二进制转十进制-8.6.vi"("子数组"=w17549) -> ("十进制数值"=w17544:i32)  [unwired: 4 out]
                    n6879 = call "数值二进制转十进制-8.6.vi"("子数组"=w17555) -> ("十进制数值"=w17543:i32)  [unwired: 4 out]
                  }
                  frame Enabled {
                    w17561 = 255 ("高字节1")
                  }
                }
                n6880 = Build Array(w17539, w17540) -> (w17542:i32[])
              }
            }
            n6881 = Insert Into Array(array=w17473, new element=w17472) -> (w17474:dbl[])  [unwired: 1 in]
          }
          n6882 = Build Array(w17467) -> (w17466:dbl[][])
        }
        frame "温度过高" {
          n6883 = Unbundle By Name(w17566) -> ("一级故障(从板)"=w17567:refnum<vi>)
          n6884 = property class="Clust (严格)"(reference=w17567) -> ("Value"=w17565:T8)  [unwired: 1 in, 2 out]
          n6885 = for {
            N: 7 -> [_]
            tunnel: w17565 -> [w17577]
            shift-right: [w17576] -> w17569
            shift-left: dbl[] [] -> [w17575]
            i -> [w17578]
            n6886 = case shown="3" w17578 {
              tunnel: w17577 -> [w17579 w17590 w17601 w17612 w17622 w17632 w17643]
              tunnel: [w17580 w17591 w17602 w17613 w17623 w17633 w17644] -> w17574
              frame 0, Default {
                # "电压过高"
                n6887 = disable-structure shown="启用" {
                  disable-tunnel: [w17586 w17589] -> w17582
                  disable-tunnel: [w17585 w17589] -> w17581
                  disable-tunnel: w17579 -> [w17584 _]
                  frame Disabled {
                    n6888 = Unbundle By Name(w17584) -> ("电压过高"=w17583:dbl)
                    n6889 = call "输入分辨率计算-EV05.vi"("1字节?"=FALSE, "数值"=w17583, "分辨率"=0.1) -> ("低字节"=w17585:dbl, "高字节1"=w17586:dbl)  [unwired: 2 in, 5 out]
                  }
                  frame Enabled {
                    w17589 = 255 ("高字节1")
                  }
                }
                n6890 = Build Array(w17582, w17581) -> (w17580:i32[])
              }
              frame 1 {
                # "电压过低"
                n6891 = disable-structure shown="启用" {
                  disable-tunnel: [w17597 w17600] -> w17593
                  disable-tunnel: [w17596 w17600] -> w17592
                  disable-tunnel: w17590 -> [w17595 _]
                  frame Disabled {
                    n6892 = Unbundle By Name(w17595) -> ("电压过低"=w17594:dbl)
                    n6893 = call "输入分辨率计算-EV05.vi"("1字节?"=FALSE, "数值"=w17594, "分辨率"=0.1) -> ("低字节"=w17596:dbl, "高字节1"=w17597:dbl)  [unwired: 2 in, 5 out]
                  }
                  frame Enabled {
                    w17600 = 255 ("高字节1")
                  }
                }
                n6894 = Build Array(w17593, w17592) -> (w17591:i32[])
              }
              frame 2 {
                # "电压不均衡"
                n6895 = disable-structure shown="启用" {
                  disable-tunnel: [w17608 w17611] -> w17604
                  disable-tunnel: [w17607 w17611] -> w17603
                  disable-tunnel: w17601 -> [w17606 _]
                  frame Disabled {
                    n6896 = Unbundle By Name(w17606) -> ("电压不均衡(V)"=w17605:dbl)
                    n6897 = call "输入分辨率计算-EV05.vi"("1字节?"=FALSE, "数值"=w17605, "分辨率"=0.1) -> ("低字节"=w17607:dbl, "高字节1"=w17608:dbl)  [unwired: 2 in, 5 out]
                  }
                  frame Enabled {
                    w17611 = 255 ("高字节1")
                  }
                }
                n6898 = Build Array(w17604, w17603) -> (w17602:i32[])
              }
              frame 3 {
                # "温度过高"
                n6899 = disable-structure shown="启用" {
                  disable-tunnel: [w17618 255 ("高字节1")] -> w17614
                  disable-tunnel: w17612 -> [w17616 _]
                  frame Enabled {
                    n6900 = Unbundle By Name(w17616) -> ("温度过高"=w17615:dbl)
                    n6901 = call "输入分辨率计算-EV05.vi"("1字节?"=TRUE, "数值"=w17615, "偏移量"=-40.0, "分辨率"=1.0) -> ("高字节1"=w17618:dbl)  [unwired: 1 in, 6 out]
                  }
                  frame Disabled {
                  }
                }
                n6902 = Build Array(w17614) -> (w17613:dbl[])
              }
              frame 4 {
                # "温度过低"
                n6903 = disable-structure shown="启用" {
                  disable-tunnel: [w17628 255 ("高字节1")] -> w17624
                  disable-tunnel: w17622 -> [w17626 _]
                  frame Disabled {
                    n6904 = Unbundle By Name(w17626) -> ("温度过低"=w17625:dbl)
                    n6905 = call "输入分辨率计算-EV05.vi"("1字节?"=TRUE, "数值"=w17625, "偏移量"=-40.0, "分辨率"=1.0) -> ("高字节1"=w17628:dbl)  [unwired: 1 in, 6 out]
                  }
                  frame Enabled {
                  }
                }
                n6906 = Build Array(w17624) -> (w17623:i32[])
              }
              frame 5 {
                # "温度不均衡"
                n6907 = disable-structure shown="启用" {
                  disable-tunnel: [w17637 255 ("高字节1")] -> w17634
                  disable-tunnel: w17632 -> [w17636 _]
                  frame Disabled {
                    n6908 = Unbundle By Name(w17636) -> ("温度不均衡"=w17635:dbl)
                    n6909 = call "输入分辨率计算-EV05.vi"("1字节?"=TRUE, "数值"=w17635, "分辨率"=1.0) -> ("高字节1"=w17637:dbl)  [unwired: 2 in, 6 out]
                  }
                  frame Enabled {
                  }
                }
                n6910 = Build Array(w17634) -> (w17633:i32[])
              }
              frame 6 {
                # "SOC过低"
                n6911 = disable-structure shown="启用" {
                  disable-tunnel: w17643 -> [w17660 _]
                  disable-tunnel: [w17646 w17663] -> w17642
                  disable-tunnel: [w17645 w17663] -> w17641
                  frame Disabled {
                    n6912 = Unbundle By Name(w17660) -> ("SOC过低"=w17659:dbl)
                    n6913 = call "输入分辨率计算-EV05.vi"("1字节?"=FALSE, "数值"=w17659, "分辨率"=0.1) -> ("低字节"=w17648:dbl, "高字节1"=w17649:dbl)  [unwired: 2 in, 5 out]
                    n6914 = call "二进制解析-8.6.vi"("索引"=4, "数值"=0) -> ("低位子数组"=w17652:i32[])  [unwired: 3 out]
                    n6915 = call "二进制解析-8.6.vi"("索引"=4, "数值"=w17649) -> ("低位子数组"=w17655:i32[])  [unwired: 3 out]
                    n6916 = call "二进制解析-8.6.vi"("索引"=4, "数值"=w17648) -> ("低位子数组"=w17653:i32[], "高位子数组"=w17654:i32[])  [unwired: 2 out]
                    n6917 = Insert Into Array(array=w17655, new element=w17654) -> (w17657:i32[])  [unwired: 1 in]
                    n6918 = Insert Into Array(array=w17653, new element=w17652) -> (w17651:i32[])  [unwired: 1 in]
                    n6919 = call "数值二进制转十进制-8.6.vi"("子数组"=w17651) -> ("十进制数值"=w17646:i32)  [unwired: 4 out]
                    n6920 = call "数值二进制转十进制-8.6.vi"("子数组"=w17657) -> ("十进制数值"=w17645:i32)  [unwired: 4 out]
                  }
                  frame Enabled {
                    w17663 = 255 ("高字节1")
                  }
                }
                n6921 = Build Array(w17641, w17642) -> (w17644:i32[])
              }
            }
            n6922 = Insert Into Array(array=w17575, new element=w17574) -> (w17576:dbl[])  [unwired: 1 in]
          }
          n6923 = Build Array(w17569) -> (w17568:dbl[][])
        }
        frame "温度过高(2)" {
          n6924 = Unbundle By Name(w17668) -> ("二级故障(从板)"=w17669:refnum<vi>)
          n6925 = property class="Clust (严格)"(reference=w17669) -> ("Value"=w17667:T8)  [unwired: 1 in, 2 out]
          n6926 = for {
            N: 7 -> [_]
            tunnel: w17667 -> [w17679]
            shift-right: [w17678] -> w17671
            shift-left: dbl[] [] -> [w17677]
            i -> [w17680]
            n6927 = case shown="3" w17680 {
              tunnel: w17679 -> [w17681 w17692 w17703 w17714 w17724 w17734 w17745]
              tunnel: [w17682 w17693 w17704 w17715 w17725 w17735 w17746] -> w17676
              frame 0, Default {
                # "电压过高"
                n6928 = disable-structure shown="启用" {
                  disable-tunnel: [w17688 w17691] -> w17684
